vi "Dictionary Test - 007.vi"(8 "error in (no error)":errorcluster) -> (0 "error out":errorcluster, 2 "pass":bool)   [LabVIEW 2009]
uses:
  <userlib>/_OpenG.lib/array/array.llb/Empty 1D Array (Variant)__ogtk.vi
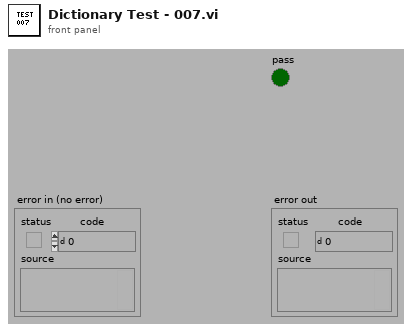
[diagram p1: front panel]
types:
  T1 = typedef "Dictionary Object RefNum.ctl" = refnum<k1>
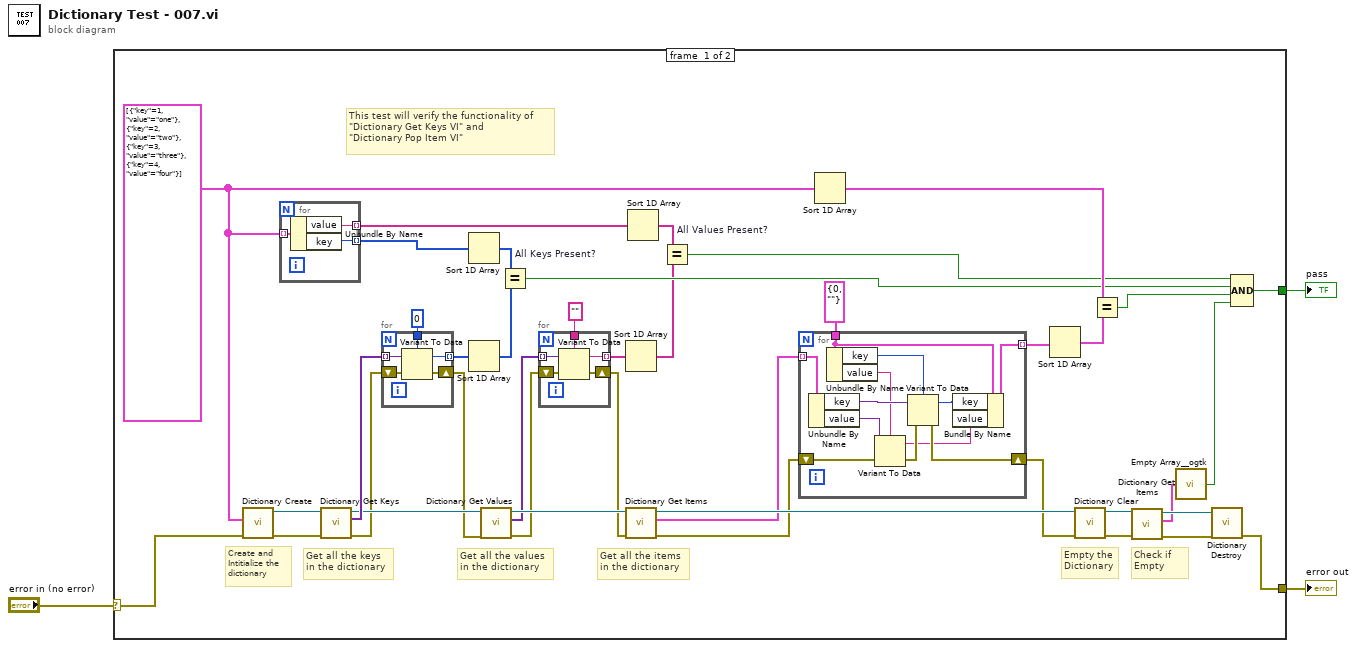
[diagram p0: block diagram]
diagram:
  n1 = case shown="No Error" "error in (no error)" {
    selector: "error in (no error)" -> [w44 w70]
    tunnel: [w43 w70] -> w1
    tunnel: [w40 _] -> w3
    frame #0 {
      w14 = cluster{"key":i32, "value":string}[] [{"key"=1, "value"="one"}, {"key"=2, "value"="two"}, {"key"=3, "value"="three"}, {"key"=4, "value"="four"}] ("dictionary with updates")
      # "Create and Intitialize the dictionary"
      # "Get all the items \nin the dictionary"
      # "Get all the values \nin the dictionary"
      # "Check if Empty"
      # "Empty the Dictionary"
      # "Get all the keys \nin the dictionary"
      # "This test will verify the functionality of \n\"Dictionary Get Keys VI\" and \n\"Dictionary Pop Item VI\""
      n2 = call "Dictionary Create.vi"("error in (no error)"=w44, "initial dictionary (empty)"=w14) -> ("error out"=w41:errorcluster, "dictionary out"=w42:T1)  [unwired: 8 in]
      n3 = for {
        tunnel: w14 -> [w69] mode=indexing
        tunnel: [w68] -> w13 mode=indexing
        tunnel: [w67] -> w11 mode=indexing
        n4 = Unbundle By Name(w69) -> ("value"=w67:string, "key"=w68:i32)
      }
      n5 = call "Dictionary Get Keys.vi"("error in (no error)"=w41, "dictionary"=w42) -> ("error out"=w26:errorcluster, "keys"=w38:variant[], "dictionary out"=w37:T1)  [unwired: 7 in]
      n6 = for {
        tunnel: w38 -> [w66] mode=indexing
        tunnel: [w65] -> w7 mode=indexing
        shift-right: [w63] -> w25
        shift-left: w26 -> [w64]
        tunnel: 0 ("key") -> [w62]
        n7 = Variant To Data(error in=w64, Variant=w66, type=w62) -> (error out=w63:errorcluster, data=w65:i32)
      }
      n8 = Sort 1D Array(array=w13) -> (sorted array=w12:i32[])
      n9 = Sort 1D Array(array=w7) -> (sorted array=w6:i32[])
      n10 = call "Dictionary Get Values.vi"("error in"=w25, "dictionary"=w37) -> ("error out"=w23:errorcluster, "values"=w22:variant[], "dictionary out"=w36:T1)  [unwired: 7 in]
      n11 = Equal? "All Keys Present?"(x=w12, y=w6) -> (x = y?=w27:bool)
      n12 = for {
        tunnel: w22 -> [w61] mode=indexing
        tunnel: [w60] -> w9 mode=indexing
        shift-right: [w58] -> w20
        shift-left: w23 -> [w59]
        tunnel: "" ("value") -> [w57]
        n13 = Variant To Data(error in=w59, Variant=w61, type=w57) -> (error out=w58:errorcluster, data=w60:string)
      }
      n14 = Sort 1D Array(array=w9) -> (sorted array=w8:string[])
      n15 = call "Dictionary Get Items.vi"("error in (no error)"=w20, "dictionary"=w36) -> ("error out"=w16:errorcluster, "items"=w19:cluster{"key":variant, "value":variant}[], "dictionary out"=w35:T1)  [unwired: 7 in]
      n16 = Sort 1D Array(array=w11) -> (sorted array=w10:string[])
      n17 = Equal? "All Values Present?"(x=w10, y=w8) -> (x = y?=w5:bool)
      n18 = for {
        tunnel: w19 -> [w56] mode=indexing
        tunnel: [w45] -> w17 mode=indexing
        tunnel: cluster{"key":i32, "value":string} {"key"=0, "value"=""} -> [w48]
        shift-right: [w50] -> w15
        shift-left: w16 -> [w49]
        n19 = Unbundle By Name(w56) -> ("key"=w54:variant, "value"=w52:variant)
        n20 = Unbundle By Name(w48) -> ("key"=w55:i32, "value"=w53:string)
        n21 = Variant To Data(error in=w49, Variant=w52, type=w53) -> (error out=w51:errorcluster, data=w46:string)
        n22 = Variant To Data(error in=w51, Variant=w54, type=w55) -> (error out=w50:errorcluster, data=w47:i32)
        n23 = Bundle By Name(cluster=w48, "key"=w47, "value"=w46) -> (w45:cluster{"key":i32, "value":string})
      }
      n24 = Sort 1D Array(array=w14) -> (sorted array=w34:cluster{"key":i32, "value":string}[])
      n25 = Sort 1D Array(array=w17) -> (sorted array=w33:cluster{"key":i32, "value":string}[])
      n26 = call "Dictionary Clear.vi"("error in (no error)"=w15, "dictionary"=w35) -> ("error out"=w31:errorcluster, "dictionary out"=w32:T1)  [unwired: 8 in]
      n27 = Equal?(x=w34, y=w33) -> (x = y?=w28:bool)
      n28 = call "Dictionary Get Items.vi"("error in (no error)"=w31, "dictionary"=w32) -> ("error out"=w29:errorcluster, "items"=w4:cluster{"key":variant, "value":variant}[], "dictionary out"=w30:T1)  [unwired: 7 in]
      n29 = call-poly <userlib>:"Empty Array__ogtk.vi"("Array"=w4) -> ("Empty Array?"=w39:bool)  [unwired: 8 in]
      n30 = call "Dictionary Destroy.vi"("error in (no error)"=w29, "dictionary"=w30) -> ("error out"=w43:errorcluster)  [unwired: 9 in]
      n31 = Compound Arithmetic op=AND(w5, w27, w28, w39) -> (w40:bool)
    }
    frame #1 {
    }
  }
  "pass" <- w3
  "error out" <- w1
